vi "AutoBike FPGA.vi"() -> ()   [LabVIEW 2016]
doc: "The roboRIO FPGA Shipping Personality. This personality supports:\n- 8 Analog Input channels with 1 sample\n- 2 Analog Output channels with 1 sample\n- 30 Digital I/O channels with 1 sample\n- 1 RSL channel\n- 4 Relay channels\n- 1 Button\n- 3 LEDs\n- 1 Accelerometer\n- 13 PWM channels\n- 6 Encoder channels\n- 2 SPI channels\n- 2 I2C channels\n- 2 UART channels\n- 1 CAN channel\n- 2 Analog Input Interrupt\n- 5 Digital Input Interrupt\n- 1 Timer Interrupt"
uses:
  Sub VIs/Utilities/Start Boolean.ctl
  <vilib>/Platform/TimedLoop/XDataNode/timing_clust.ctl
  <vilib>/Platform/TimedLoop/XDataNode/nitl_modes.ctl
  <vilib>/Platform/TimedLoop/XDataNode/wakeup.ctl
  <vilib>/rvi/Emulation/niFpgaGetClockAttributes.vi
  <vilib>/rvi/Emulation/niFpgaSctlEmulationGetInTimedLoop.vi
  <vilib>/rvi/Emulation/niFpgaEmulationReportErrorSimple.vi
  <vilib>/rvi/eio/common/nirviEmuTemplateMethod_errors.vi
  <vilib>/rvi/Emulation/niFpgaCriticalErrorInLSC.vi
  <vilib>/rvi/Emulation/niFpgaProcessEmulError.vi
  <vilib>/rvi/Emulation/niFpgaEmulationIsFPGAContextNoSignature.vi
  <vilib>/rvi/errors/niFpgaSetErrorForExecOnDevCompSimple.vi
  <vilib>/rvi/eio/common/nirviEmuReportErrorAndStop.vi
  <vilib>/rvi/DataTransferAndStorage/Container/Common/niFpgaContainerGetUniqueNameForEmu.vi
  <vilib>/rvi/FIFO/Fifo_Resource/nirvififoEmulationSetSize.vi
  <vilib>/rvi/FIFO/Fifo_Resource/nirviFifoEmulationQueueMgr.vi
  <instcachedir>/0/nirviFifoEmulationQueueMgr_E5CAEC123FF24DC58D834DCA3CDAA9B5.lvgen/nirviFifoEmulationQueueMgr_E5CAEC123FF24DC58D834DCA3CDAA9B5_002.vi
  <vilib>/Utility/error.llb/Clear Errors.vi
  <vilib>/rvi/FIFO/Fifo_Resource/nirvififoEmulationCreateLock.vi
  <vilib>/rvi/FIFO/Fifo_Resource/nirvififoEmulationObtainLock.vi
  <vilib>/rvi/FIFO/Fifo_Resource/nirvififoEmulationReleaseLock.vi
  <vilib>/rvi/occurrence/nirviWaitOnOccurrenceBase.vi
  <vilib>/rvi/errors/nirviReportUnexpectedCaseInternalError.vi
  <vilib>/rvi/errors/nirviReportUnexpectedCaseInternalError (U32).vi
  <vilib>/rvi/FIFO/Fifo_Resource/nirvififoEmulationDetermineInputValidOut.vi
  <vilib>/rvi/DataTransferAndStorage/Container/Common/niFpgaContainerSetEmuInfo.vi
  <vilib>/eio/EIONode/EIONode.xnode
  <vilib>/rvi/DataTransferAndStorage/Container/XNode/niFpgaContainer.xnode
  <vilib>/rvi/FIFO/Fifo_Resource/nirvififoEmulationRead.vi
  <vilib>/rvi/FIFO/Fifo_Resource/nirvififoEmulationWrite.vi
  <vilib>/platform/TimedLoop/XDataNode/XDataNode.xnode
  <vilib>/rvi/LocalResourceManager/LocalResourceManager.xnode
  <vilib>/Platform/TimedLoop/XDataNode/XDNodeRunTimeDep.lvlib
panel:
  in  "Freq":u32 caption="Count(Ticks)"
  in  "Control Loop Duty Cycle":sgl
  in  "Control Loop Direction":bool
  in  "Front Panel Duty Cycle":sgl
  in  "Front Panel Direction":bool
  in  "Shut Down BW":bool
  out "Duty cycle (steering)":sgl
  out "Steering angle(deg)":sgl
  in  "Duty Cycle in":sgl
  in  "Count(uSec)":u32=1
  out "Current velocity":sgl
  out "Duty cycle (BW)":sgl
  in  "Reference velocity in km/h":sgl=15.0
  out "Filtered data":i32
  out "Value Channel 0":i32
  out "Channel 4 position":i32
  out "Channel 5 position":i32
  out "Channel 6 position":i32
  out "Channel 7 position":i32
  out "Position":i64
  in  "Stop encoder":bool
  in  "Reset counter":bool
  in  "Stop direction switch":bool
  in  "Switch direction":bool
  out "HallSensorValue":u8
  in  "Stop Hallsensor":bool
  out "dt":u32
  out "DIO.SPI_CS3:0.IN":u8 format="%08b"
  in  "DIO.SPI_CS3:0.DIR":u8 format="%08b"
  in  "DIO.SPI_CS3:0.OUT":u8 format="%08b"
  in  "IRQ.TIMER.SETTIME":T1
  in  "IRQ.TIMER.WRITE":u32
  out "IRQ.TIMER.READ":u32
  in  "IRQ.DI_BTN.NO":u8
  in  "IRQ.DI_BTN.CNT":u32
  in  "IRQ.DI_BTN.FALL":bool
  in  "IRQ.DI_BTN.RISE":bool
  in  "IRQ.DI_BTN.ENA":bool
  in  "IRQ.AI_B_0.HYSTERESIS":u16=17
  in  "IRQ.AI_B_1.HYSTERESIS":u16=17
  in  "IRQ.AI_B_1.NO":u8
  in  "IRQ.AI_B_0.NO":u8
  in  "IRQ.AI_B_1.THRESHOLD":u16
  in  "IRQ.AI_B_0.THRESHOLD":u16
  in  "IRQ.AI_B_3:0.CNFG":u8 format="%.0b"
  in  "IRQ.DIO_B_0.NO":u8
  in  "IRQ.DIO_B_1.NO":u8
  in  "IRQ.DIO_B_2.NO":u8
  in  "IRQ.DIO_B_3.NO":u8
  in  "IRQ.DIO_B_3.CNT":u32
  in  "IRQ.DIO_B_2.CNT":u32
  in  "IRQ.DIO_B_1.CNT":u32
  in  "IRQ.DIO_B_0.CNT":u32
  in  "IRQ.DIO_B_7:0.FALL":u8 format="%08b"
  in  "IRQ.DIO_B_7:0.RISE":u8 format="%08b"
  in  "IRQ.DIO_B_7:0.ENA":u8 format="%08b"
  in  "SPI.SPI.IRQ.NO":u8=15
  in  "SPI.B.IRQ.NO":u8=15
  out "DIO.DIO_9:8.IN":u8 format="%08b"
  in  "ENC.DIO_3.CNFG":u8 format="%08b"
  out "ENC.DIO_3.CNTR":u32
  out "ENC.DIO_3.STAT":u8 format="%08b"
  in  "ENC.DIO_4.CNFG":u8 format="%08b"
  out "ENC.DIO_4.CNTR":u32
  out "ENC.DIO_4.STAT":u8 format="%08b"
  in  "DIO.DIO_9:8.OUT":u8 format="%08b"
  in  "DIO.DIO_9:8.DIR":u8 format="%08b"
  in  "ENC.DIO_2.CNFG":u8 format="%08b"
  out "ENC.DIO_2.CNTR":u32
  out "ENC.DIO_2.STAT":u8 format="%08b"
  out "ENC.DIO_1.STAT":u8 format="%08b"
  out "ENC.DIO_1.CNTR":u32
  in  "ENC.DIO_1.CNFG":u8 format="%08b"
  out "DIO.DIO_7:0.IN":u8 format="%08b"
  in  "SYS.SELECTDIO":u8 format="%08b"
  in  "DIO.DIO_7:0.DIR":u8 format="%08b"
  in  "DIO.DIO_7:0.OUT":u8 format="%08b"
  out "ENC.DIO_0.STAT":u8 format="%08b"
  out "ENC.DIO_0.CNTR":u32
  in  "ENC.DIO_0.CNFG":u8 format="%08b"
  out "DI.BTN":u8 format="%08b"
  in  "DO.LED 5:0":u8 format="%06b"
  in  "DO.RSL.OUT":bool
  out "SPI.SPI.STAT":u8 format="%08b"
  in  "SPI.SPI.GO":T1
  in  "SPI.SPI.CNT":u16
  in  "SPI.SPI.CNFG":u16 format="%016b"
  out "SPI.SPI.DATI":u16
  in  "SPI.SPI.DATO":u16
  out "I2C.I2C.DATI":u8
  out "I2C.I2C.STAT":u8 format="%08b"
  in  "I2C.I2C.DATO":u8
  in  "I2C.I2CADDR":u8 format="%08b"
  in  "I2C.I2C.CNTR":u8
  in  "I2C.I2C.CNTL":u8 format="%08b"
  in  "I2C.I2C.CNFG":u8 format="%08b"
  in  "I2C.I2C.GO":T1
  out "ACC.Z.VAL":u16
  out "ACC.Y.VAL":u16
  out "ACC.X.VAL":u16
  in  "DO.RELAY.OUT":u8 format="%08b"
  out "SYS.ACC.RDY":bool
  out "SYS.RDY":bool
  in  "PWM.PWM_5.MAX":u16
  in  "PWM.PWM_5.CMP":u16
  in  "PWM.PWM_5.CNFG":u8 format="%08b"
  in  "PWM.PWM_5.CS":u8
  out "PWM.PWM_5.CNTR":u16
  in  "PWM.PWM_6.MAX":u16
  in  "PWM.PWM_6.CMP":u16
  in  "PWM.PWM_6.CNFG":u8 format="%08b"
  in  "PWM.PWM_6.CS":u8
  out "PWM.PWM_6.CNTR":u16
  in  "PWM.PWM_7.MAX":u16
  in  "PWM.PWM_7.CMP":u16
  in  "PWM.PWM_7.CNFG":u8 format="%08b"
  in  "PWM.PWM_7.CS":u8
  out "PWM.PWM_7.CNTR":u16
  in  "PWM.PWM_8.MAX":u16
  in  "PWM.PWM_8.CMP":u16
  in  "PWM.PWM_8.CNFG":u8 format="%08b"
  in  "PWM.PWM_8.CS":u8
  out "PWM.PWM_8.CNTR":u16
  in  "PWM.PWM_9.MAX":u16
  in  "PWM.PWM_9.CMP":u16
  in  "PWM.PWM_9.CNFG":u8 format="%08b"
  in  "PWM.PWM_9.CS":u8
  out "PWM.PWM_9.CNTR":u16
  in  "PWM.PWM_4.MAX":u16
  in  "PWM.PWM_4.CMP":u16
  in  "PWM.PWM_4.CNFG":u8 format="%08b"
  in  "PWM.PWM_4.CS":u8
  out "PWM.PWM_4.CNTR":u16
  in  "PWM.PWM_3.MAX":u16
  in  "PWM.PWM_3.CMP":u16
  in  "PWM.PWM_3.CNFG":u8 format="%08b"
  in  "PWM.PWM_3.CS":u8
  out "PWM.PWM_3.CNTR":u16
  in  "PWM.PWM_2.MAX":u16
  in  "PWM.PWM_2.CMP":u16
  in  "PWM.PWM_2.CNFG":u8 format="%08b"
  in  "PWM.PWM_2.CS":u8
  out "PWM.PWM_2.CNTR":u16
  in  "PWM.PWM_1.MAX":u16
  in  "PWM.PWM_1.CMP":u16
  in  "PWM.PWM_1.CNFG":u8 format="%08b"
  in  "PWM.PWM_1.CS":u8
  out "PWM.PWM_1.CNTR":u16
  out "PWM.PWM_0.CNTR":u16
  in  "PWM.PWM_0.CS":u8
  in  "PWM.PWM_0.CNFG":u8 format="%08b"
  in  "PWM.PWM_0.CMP":u16
  in  "PWM.PWM_0.MAX":u16
  in  "AO.B_0.VAL":u16
  in  "AO.B_1.VAL":u16
  in  "AO.SYS.GO":T1
  out "AO.SYS.STAT":bool
  out "AI.B_0.VAL":u16
  out "AI.B_1.VAL":u16
  out "AI.B_2.VAL":u16
  out "AI.B_3.VAL":u16
  out "AI.AI_0.VAL":u16
  out "AI.AI_1.VAL":u16
  out "AI.AI_2.VAL":u16
  out "AI.AI_3.VAL":u16
  out "SYS.AI.RDY":bool
  in  "SYS.SELECTB":u8 format="%08b"
  in  "DIO.B_7:0.OUT":u8 format="%08b"
  in  "DIO.B_7:0.DIR":u8 format="%08b"
  out "DIO.B_7:0.IN":u8 format="%08b"
  in  "DIO.B_15:8.OUT":u8 format="%08b"
  in  "DIO.B_15:8.DIR":u8 format="%08b"
  out "DIO.B_15:8.IN":u8 format="%08b"
  in  "SPI.B.DATO":u16
  out "SPI.B.DATI":u16
  in  "SPI.B.CNFG":u16 format="%016b"
  in  "SPI.B.CNT":u16
  in  "SPI.B.GO":T1
  out "SPI.B.STAT":u8 format="%08b"
  in  "PWM.B_0.MAX":u16
  in  "PWM.B_0.CMP":u16
  in  "PWM.B_0.CNFG":u8 format="%08b"
  in  "PWM.B_0.CS":u8
  out "PWM.B_0.CNTR":u16
  in  "PWM.B_1.CMP":u16
  in  "PWM.B_1.MAX":u16
  out "PWM.B_1.CNTR":u16
  in  "PWM.B_1.CNFG":u8 format="%08b"
  in  "PWM.B_1.CS":u8
  in  "PWM.B_2.CMP":u16
  in  "PWM.B_2.MAX":u16
  out "PWM.B_2.CNTR":u16
  in  "PWM.B_2.CNFG":u8 format="%08b"
  in  "PWM.B_2.CS":u8
  in  "I2C.B.DATO":u8
  out "I2C.B.DATI":u8
  in  "I2C.B.ADDR":u8 format="%08b"
  in  "I2C.B.CNTR":u8
  in  "I2C.B.CNTL":u8 format="%08b"
  out "I2C.B.STAT":u8 format="%08b"
  in  "I2C.B.CNFG":u8 format="%08b"
  in  "I2C.B.GO":T1
  in  "ENC.B.CNFG":u8 format="%08b"
  out "ENC.B.CNTR":u32
  out "ENC.B.STAT":u8 format="%08b"
  # "System"
  # "Onboard Devices"
  # "Connector B"
  # "DIO"
  # "SPI"
  # "PWM"
  # "I2C"
  # "AI"
  # "RELAY"
  # "RSL"
  # "Accelerometer"
  # "SPI Master"
  # "Analog Input"
  # "Analog Output"
  # "Digital I/O"
  # "Counters / PWM"
  # "Digital I/O"
  # "Encoders"
  # "IO Configuration"
  # "Buttons & LEDs"
  # "SPI CS DIO"
  # "Analog Interrupt"
  # "Digital Interrupt"
  # "Encoders"
  # "IO Configuration"
  # "Button Interrupt"
  # "I2C Master"
  # "FPGA Timer"
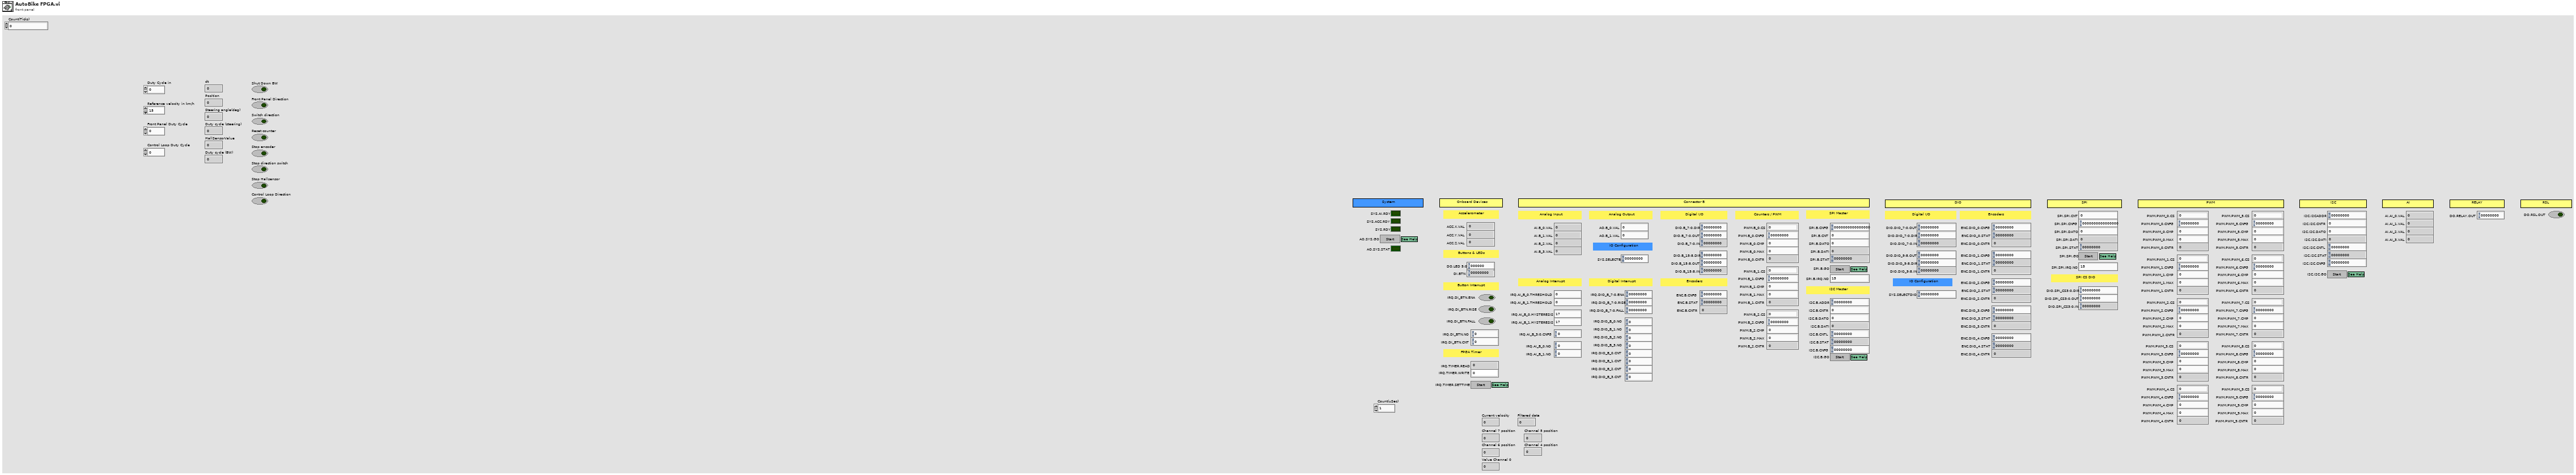
[diagram p1: front panel]
types:
  T1 = typedef "Start Boolean.ctl" = bool
  T2 = typedef "XDNodeRunTimeDep.lvlib/timing_clust.ctl" = cluster{"Expected End [f-1]":u64, "Actual End [f-1]":u64, "Finished Late? [f-1]":bool, "Expected End [i-1]":u64, "Actual End [i-1]":u64, "Finished Late? [i-1]":bool, "Expected Start [i]":u64, "Actual Start [i]":u64, "Expected Start [f]":u64, "Actual Start [f]":u64, "Source Name":string, "Structure Name":string, "Period":i64, "Deadline":i64, "Offset":i64, "Start":i64, "Priority":i32, "Timeout":i32, "Mode":T3, "Wakeup Reason":T4, "Error":errorcluster, "Source Type":string, "Secondary Source Type":string, "Global End Time":u64, "Global Start Time":u64, "Frame Duration":u64, "Iteration Duration":u64, "Assigned CPU":i32, "I/O Scan Engine Mode":u32}
  T3 = typedef "XDNodeRunTimeDep.lvlib/nitl_modes.ctl" = enum32{"No Change", "Process missed periods, maintain original phase", "Discard missed periods, maintain original phase", "Process missed periods, ignore original phase", "Discard missed periods, ignore original phase"}
  T4 = typedef "XDNodeRunTimeDep.lvlib/wakeup.ctl" = enum32{"Normal", "Aborted", "Asynchronous wakeup", "Timing source error", "Timed loop error", "Timeout"}
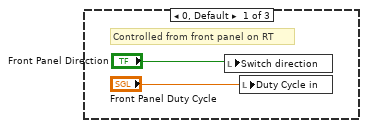
[diagram p2: hidden frame]
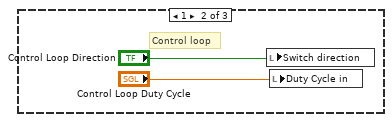
[diagram p3: hidden frame]
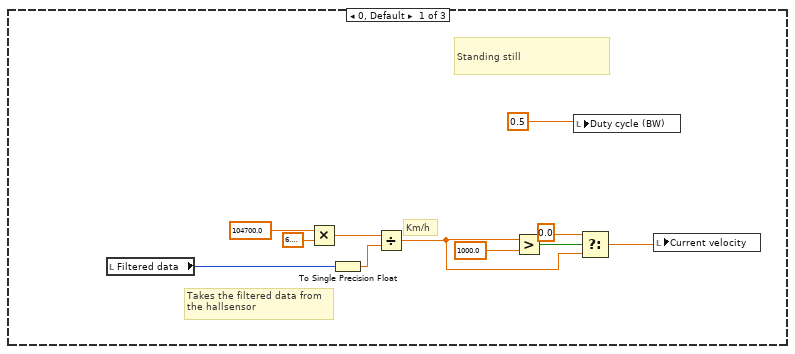
[diagram p4: hidden frame]
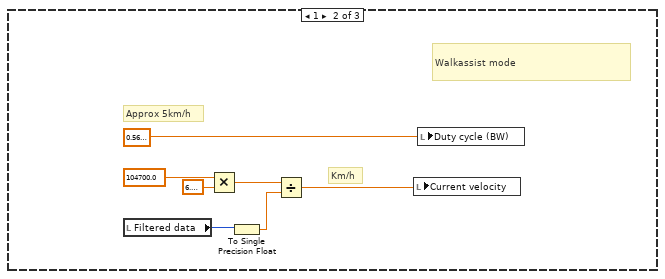
[diagram p5: hidden frame]
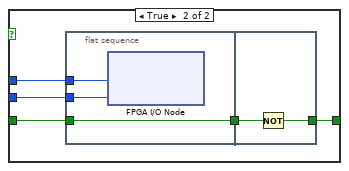
[diagram p12: hidden frame]
diagram:
  # "DONT USE PWN 1, IT IS CONNECTED ON THREE OUTS"
  # "The accelerometer nodes take some time before the FPGA can first read the values. This is because it takes time to read from the accelerometer. An iteration of the While Loop will not complete until the accelerometer values have been read.\n\nAfter the completion of the first iteration of the While Loop, all indicators have valid values."
  # "The analog output nodes take some time before the FPGA write the values to the pins. The GO and STAT registers are used to handshake between the FPGA and host. When the host wants the values to be written, the host sets the GO register to TRUE. If the host reads the STAT register before setting the value of the GO register, it can wait for the value of the STAT register to invert. The value inversion tells the host that the output values have been written."
  # "The FPGA timer fires the interrupt request (IRQ) when TIMER.Read counts down to zero. If TIMER.Read is not zero, it counts down to one per microsecond."
  # "The analog input nodes take some time before the FPGA can first read the values. This is because it takes time to set up the Analog-to-Digital converter (ADC) and convert the first reading. An iteration of the While Loop will not complete until all the analog input channels have been sampled.\n\nAfter the completion of the first iteration of the While Loop, all indicators have valid values."
  # "Note: On some hardware a \"ghosting effect\" may occur on any unconnected AI channels. For example, if channel AI0 is connected and channels AI1~AI7 are not connected the the value read at AI0 may be seen on indicators AI1~AI7. This is common for hardware that use a multiplexed (MUXed) Analog-to-Digital converter (ADC), because the input analog signal is used to charge a capacitor which does not discharge before the unconnected channel is read.\n\nYou can hide the \"ghosting effect\" by using an mask register. This register is used to decide when the indicator should be updated."
  # "The only interface that sends interrupts to the RT side. Timer interrupts, analog input interrupts, digital input interrupts, and SPI interrupt share this interface.\n\nAll interrupts work in sequence. One interrupt waits until the previous interrupt request (IRQ) gets acknowledged on the RT side."
  # "NOTE: The SYS.RDY boolean MUST exist and must become TRUE at some point otherwise the myRIO API will not function correctly."
  # "There is some delay between when the FPGA code starts and the analog inputs, accelerometer, and scaling values outputs are valid. If the host wants to ensure that there are valid values in theses registers it should wait for each subsystem to finish its initialization process. \n\nWhen all subsystems have finished initializinig, the SYS.RDY indicator will be true, which can be polled by the host to determine the status of the FPGA. Alternatively, the host can poll the individual SYS.xx.RDY indicators to determine the status of the individual subsystems.\n\nThis loop continues indefinitely, essentially making SYS.RDY a read-only register."
  n1 = flat-sequence {
    tunnel: [i64 0] -> w2
    tunnel: [TRUE ("DIO/DIO3")] -> w1
    tunnel: w2 -> [w29]
    tunnel: w1 -> [w28]
    frame #0 {
      # "Initialise"
    }
    frame #1 {
      n2 = while {
        shift-right: [w49] -> _
        shift-left: w28 -> [w51]
        stop <- "Stop Hallsensor" stop-if-true
        n3 = flat-sequence {
          tunnel: w51 -> [w54]
          tunnel: [w54] -> w48
          tunnel: [u8 0] -> w47
          tunnel: [w52] -> w46
          tunnel: w48 -> [w59]
          tunnel: w47 -> [w57]
          tunnel: w46 -> [w56]
          tunnel: [w58] -> w45
          tunnel: [w55] -> w44
          tunnel: [w81] -> w49
          tunnel: w45 -> [w81]
          tunnel: [w80] -> w43
          tunnel: w44 -> [w78]
          frame #0 {
            n4 = call "Tick Count4"() -> ("Tick Count(uSec)"=w52:u32)
          }
          frame #1 {
            n5 = node-c288() -> (w61:T2)  [unwired: 1 in]
            n6 = timed-loop {
              shift-right: [w65] -> _
              shift-left: w57 -> [w62]
              shift-right: [w70] -> w58
              shift-left: w59 -> [w73]
              timing: w61 -> [_]
              timing-out: [_] -> w60
              tunnel: w56 -> [w72]
              tunnel: [w72] -> w55
              stop <- w64 stop-if-true
              # "Calculates the time it takes to collect 2 rises, i.e one magnet"
              # "Reads the output from the hallsensor and outputs the number of change in rises"
              # "Hallsensor counter"
              n7 = xnode "FPGA I/O Node"() -> ("DIO/DIO8"=w70:bool)  [unwired: 1 in, 1 out]
              n8 = Exclusive Or(1:w73, 2:w70) -> (0:w68:bool)
              n9 = Not And(1:TRUE ("y"), 2:w70) -> (0:w69:bool)
              n10 = And(x=w69, y=w68) -> (x .and. y?=w67:bool)
              n11 = Increment(x=w62) -> (x+1=w66:u8)
              n12 = Select(t=w66, s=w67, f=w62) -> (s? t:f=w65:u8)
              "HallSensorValue" <- w65
              n13 = Equal?(x=u8 2, y=w65) -> (x = y?=w64:bool)
            }
            n14 = node-c288(w60) -> ()
          }
          frame #2 {
            n15 = call "Tick Count"() -> ("Tick Count(uSec)"=w79:u32)
            n16 = Subtract(x=w79, y=w78) -> (x-y=w80:u32)
          }
        }
        n17 = To Long Integer(number=w43) -> (32bit integer=w42:i32)
        n18 = call "Median filter.vi"("Rawdata"=w42) -> ("Filtered element"=w39:i32)  [unwired: 10 in]
        n19 = Equal To 0?(x=w39) -> (x = 0?=w41:bool)
        n20 = Select(t=1, s=w41, f=w39) -> (s? t:f=→"Filtered data":i32)
      }
      n21 = node-c288() -> (w31:T2)  [unwired: 1 in]
      n22 = node-c288() -> (w27:T2)  [unwired: 1 in]
      n23 = timed-loop {
        shift-right: [w92] -> _
        shift-left: w29 -> [w83]
        shift-right: [w89] -> _
        shift-left: _ -> [w87]
        shift-right: [w88] -> _
        shift-left: _ -> [w86]
        timing: w31 -> [_]
        timing-out: [_] -> w30
        stop <- "Stop encoder" stop-if-true
        # "Decoder, reads both signals and check if there is any change to any of the channels, if there is a change current A channel\nis compared to previous B channel to determine which direction the motor is going and updates the position counter\naccordingly. The counter is resetted each time the Main VI is deployed."
        # "Motor Decoder"
        n24 = xnode "FPGA I/O Node"() -> ("DIO/DIO0"=w89:bool, "DIO/DIO1"=w88:bool)  [unwired: 2 in, 2 out]
        n25 = Exclusive Or(1:w86, 2:w89) -> (0:w85:bool)
        n26 = Select(t=i64 0, s="Reset counter", f=w83) -> (s? t:f=w91:i64)
        n27 = Exclusive Or(1:w87, 2:w89) -> (0:w99:bool)
        n28 = Exclusive Or(1:w86, 2:w88) -> (0:w98:bool)
        n29 = Or(x=w99, y=w98) -> (x .or. y?=w84:bool)
        n30 = Select(t=i64 1, s=w85, f=i64 -1) -> (s? t:f=w94:i64)
        n31 = Add(x=w94, y=w91) -> (x+y=w93:i64)
        n32 = Select(t=w93, s=w84, f=w91) -> (s? t:f=w92:i64)
        "Position" <- w92
      }
      n33 = timed-loop {
        timing: w27 -> [_]
        timing-out: [_] -> w26
        stop <- "Stop direction switch" stop-if-true
        # "Switch the direction of the steering\nmotor."
        # "Switch direction"
        n34 = xnode "FPGA I/O Node"("DIO/DIO2"="Switch direction") -> ()  [unwired: 1 in, 1 out]
      }
      n35 = node-c288(w26) -> ()
      n36 = node-c288(w30) -> ()
    }
  }
  n37 = while {
    stop <- FALSE stop-if-true
    # "PWM signal to steering motor"
    n38 = flat-sequence {
      tunnel: ["Freq"] -> w104
      tunnel: [w112] -> w106
      tunnel: w104 -> [w109]
      tunnel: w106 -> [w114]
      frame #0 {
        # "2000 ticks=20 000Hz"
        n39 = call "Loop Timer3"("Count(Ticks)"="Freq") -> ()  [unwired: 1 out]
      }
      frame #1 {
        n40 = local read "Duty cycle (steering)"() -> (w110:sgl)
        n41 = To Single Precision Float(number=w109) -> (single precision float=w108:sgl)
        n42 = Not Equal To 0?(x=w110) -> (x != 0?=w111:bool)
        n43 = Multiply(x=w110, y=w108) -> (x*y=w113:sgl)
        n44 = xnode "FPGA I/O Node"("PWM/PWM0"=w111) -> ()  [unwired: 1 in, 1 out]
        n45 = To Unsigned Long Integer(number=w113) -> (unsigned 32bit integer=w112:u32)
      }
      frame #2 {
        n46 = call "Wait3"("Count(Ticks)"=w114) -> ()  [unwired: 1 out]
      }
      frame #3 {
        n47 = xnode "FPGA I/O Node"("PWM/PWM0"=FALSE ("PWM/PWM8")) -> ()  [unwired: 1 in, 1 out]
      }
    }
  }
  n48 = while {
    stop <- FALSE stop-if-true
    # "Backwheel motor control"
    n49 = local read "Channel 5 position"() -> (w116:i32)
    n50 = case shown="2" w116 {
      frame 0, Default {
        # "Takes the filtered data from\nthe hallsensor"
        # "Km/h"
        # "Standing still"
        n51 = local read "Filtered data"() -> (w119:i32)
        n52 = Multiply(x=sgl 104700.0, y=sgl 6.2831855) -> (x*y=w125:sgl)
        n53 = To Single Precision Float(number=w119) -> (single precision float=w120:sgl)
        n54 = Divide(x=w125, y=w120) -> (x/y=w121:sgl)
        n55 = Greater?(x=w121, y=sgl 1000.0) -> (0:w123:bool)
        n56 = local write "Duty cycle (BW)"(sgl 0.5 ("Duty cycle out 2")) -> ()
        n57 = Select(t=sgl 0.0, s=w123, f=w121) -> (s? t:f=w118:sgl)
        n58 = local write "Current velocity"(w118) -> ()
      }
      frame 1 {
        # "Walkassist mode"
        # "Approx 5km/h"
        # "Km/h"
        n59 = local read "Filtered data"() -> (w132:i32)
        n60 = Multiply(x=sgl 104700.0, y=sgl 6.2831855) -> (x*y=w133:sgl)
        n61 = To Single Precision Float(number=w132) -> (single precision float=w131:sgl)
        n62 = Divide(x=w133, y=w131) -> (x/y=w130:sgl)
        n63 = local write "Current velocity"(w130) -> ()
        n64 = local write "Duty cycle (BW)"(sgl 0.56 ("Duty cycle out")) -> ()
      }
      frame 2 {
        n65 = while {
          shift-right: [w141] -> _
          shift-left: sgl 0.56 -> [w144]
          stop <- w138 stop-if-true
          # "This is in case we are starting from\nstanding still and we try to divide with 0, \nwhich will give us an inf value."
          # "Cruise control"
          # "Takes the filtered data from\nthe hallsensor"
          # "Wheel radius=0.349m\nnumber of magnets=12\nFormulas:\ndt/1 000 000 * number of magnets = time between magnets\nDivide wheel circumfence with time between two magnets multiplied\n by number of magnets, multiplied by 3.6 to get it in km/h.\n\n(2pi(0.349*1 000 000*3.6/12)) / dt = km/h"
          # "Km/h"
          n66 = local read "Filtered data"() -> (w150:i32)
          n67 = Multiply(x=sgl 104700.0, y=sgl 6.2831855) -> (x*y=w156:sgl)
          n68 = To Single Precision Float(number=w150) -> (single precision float=w151:sgl)
          n69 = Divide(x=w156, y=w151) -> (x/y=w152:sgl)
          n70 = Greater?(x=w152, y=sgl 1000.0) -> (0:w154:bool)
          n71 = Select(t=sgl 0.0, s=w154, f=w152) -> (s? t:f=w137:sgl)
          "Current velocity" <- w137
          n72 = Less Or Equal?(x=w137, y="Reference velocity in km/h") -> (x <= y?=w142:bool)
          n73 = Add(x=sgl 1e-06 ("y"), y=w144) -> (x+y=w145:sgl)
          n74 = Subtract(x=w144, y=sgl 1e-06) -> (x-y=w146:sgl)
          n75 = local read "Channel 5 position"() -> (w140:i32)
          n76 = Select(t=w145, s=w142, f=w146) -> (s? t:f=w141:sgl)
          "Duty cycle (BW)" <- w141
          n77 = call "Wait"("Count(uSec)"="Count(uSec)") -> ()  [unwired: 1 out]
          n78 = Not Equal?(x=w140, y=2) -> (x != y?=w138:bool)
        }
      }
    }
  }
  n79 = while {
    stop <- FALSE stop-if-true
    # "PWM signal to backwheel motor"
    n80 = flat-sequence {
      tunnel: [w164] -> w160
      tunnel: w160 -> [w167]
      frame #0 {
        # "80 000ticks=500Hz"
        n81 = call "Loop Timer2"("Count(Ticks)"=u32 80000) -> ()  [unwired: 1 out]
      }
      frame #1 {
        n82 = local read "Duty cycle (BW)"() -> (w162:sgl)
        n83 = xnode "FPGA I/O Node"("PWM/PWM8"=TRUE) -> ()  [unwired: 1 in, 1 out]
        n84 = Multiply(x=w162, y=sgl 80000.0) -> (x*y=w165:sgl)
        n85 = To Unsigned Long Integer(number=w165) -> (unsigned 32bit integer=w164:u32)
      }
      frame #2 {
        n86 = call "Wait2"("Count(Ticks)"=w167) -> ()  [unwired: 1 out]
      }
      frame #3 {
        n87 = xnode "FPGA I/O Node"("PWM/PWM8"=FALSE) -> ()  [unwired: 1 in, 1 out]
      }
    }
  }
  n88 = while {
    stop <- FALSE stop-if-true
    # "Host Synchronization"
    n89 = local read "SYS.ACC.RDY"() -> (w170:bool)
    n90 = local read "SYS.AI.RDY"() -> (w172:bool)
    n91 = Compound Arithmetic op=AND(w172, w170) -> (→"SYS.RDY":bool)
  }
  n92 = while {
    stop <- FALSE stop-if-true
    # "Interrupt to RT"
    n93 = xnode ("FIFO Method Node")("Timeout"=-1) -> ("Element"=w175:u8)  [unwired: 1 in, 2 out]
    n94 = call <vilib>:"niFPGA Interrupt.vi"("Wait Until Cleared (F)"=TRUE, "IRQ Number (0)"=w175) -> ()  [unwired: 1 in]
  }
  n95 = while {
    stop <- FALSE stop-if-true
    # "Steering motor"
    n96 = local read "Switch direction"() -> (w182:bool)
    n97 = local read "Position"() -> (w179:i64)
    n98 = call "Steering motor.vi"("Steering position (in pulses)"=w179, "Duty Cycle in"="Duty Cycle in", "Switch direction"=w182) -> ("Duty Cycle out"=→"Duty cycle (steering)":sgl, "Steering angle(deg)"=→"Steering angle(deg)":sgl)  [unwired: 7 in]
  }
  n99 = while {
    stop <- FALSE stop-if-true
    # "Receiver"
    n100 = call "Receiver.vi"() -> ("Channel 7 position"=→"Channel 7 position":i32, "Channel 6 position"=→"Channel 6 position":i32, "Channel 5 position"=w186:i32, "Channel 4 position"=→"Channel 4 position":i32, "Value Channel 0"=→"Value Channel 0":i32)  [unwired: 7 in]
    n101 = Select(t=0, s="Shut Down BW", f=w186) -> (s? t:f=→"Channel 5 position":i32)
  }
  n102 = while {
    stop <- FALSE stop-if-true
    # "RC steering motor switch"
    n103 = local read "Channel 6 position"() -> (w193:i32)
    n104 = case shown="2" w193 {
      frame 0, Default {
        # "Controlled from front panel on RT"
        n105 = local write "Switch direction"("Front Panel Direction") -> ()
        n106 = local write "Duty Cycle in"("Front Panel Duty Cycle") -> ()
      }
      frame 1 {
        # "Control loop"
        n107 = local write "Switch direction"("Control Loop Direction") -> ()
        n108 = local write "Duty Cycle in"("Control Loop Duty Cycle") -> ()
      }
      frame 2 {
        n109 = local read "Value Channel 0"() -> (w200:i32)
        n110 = call "RC steering motor interpolation.vi"("Value Channel 0"=w200) -> ("Numeric"=w199:sgl, "Boolean"=w198:bool)  [unwired: 9 in]
        n111 = local write "Duty Cycle in"(w199) -> ()
        n112 = local write "Switch direction"(w198) -> ()
      }
    }
  }
  n113 = while {
    stop <- FALSE stop-if-true
    # "Timer"
    n114 = local read "IRQ.TIMER.READ"() -> (w204:u32)
    n115 = Select(t="IRQ.TIMER.WRITE", s="IRQ.TIMER.SETTIME", f=w204) -> (s? t:f=w202:u32)
    n116 = case shown="Default" w202 {
      selector: w202 -> [w208 w211]
      tunnel: [w208 w209] -> w201
      frame 0 {
      }
      frame Default {
        n117 = Decrement(x=w211) -> (x-1=w210:u32)
        n118 = case shown="0" w210 {
          selector: w210 -> [w212 w215]
          tunnel: [w212 w215] -> w209
          frame Default {
          }
          frame 0 {
            w214 = u8 0  # Reserved for Timer IRQ
            n119 = xnode ("FIFO Method Node")("Element"=w214, "Timeout"=-1) -> ()  [unwired: 1 in, 2 out]
          }
        }
      }
    }
    "IRQ.TIMER.READ" <- w201
    n120 = call "Loop Timer"("Count(uSec)"=u8 1 ("Count(mSec)")) -> ()  [unwired: 1 out]
  }
  n121 = xnode "VI-Defined FIFO Configuration"() -> ("FIFO Out"=w4:refnum<k21>)
  n122 = while {
    tunnel: w4 -> [w224]
    i -> [w238]
    stop <- FALSE stop-if-true
    # "Analog Input"
    n123 = Greater Than 0?(x=w238) -> (x > 0?=→"SYS.AI.RDY":bool)
    n124 = xnode "FPGA I/O Node"() -> ("MXP/AI0"=w217:u16, "MXP/AI1"=w216:u16, "MXP/AI2"=→"AI.B_2.VAL":u16, "MXP/AI3"=→"AI.B_3.VAL":u16, "AnalogIn0"=→"AI.AI_0.VAL":u16, "AnalogIn1"=→"AI.AI_1.VAL":u16, "AnalogIn2"=→"AI.AI_2.VAL":u16, "AnalogIn3"=→"AI.AI_3.VAL":u16)  [unwired: 8 in, 8 out]
    "AI.B_0.VAL" <- w217
    "AI.B_1.VAL" <- w216
    n125 = Number To Boolean Array(number="IRQ.AI_B_3:0.CNFG") -> (Boolean array=w225:bool[])
    n126 = Index Array(array=w225) -> (element #1=w227:bool, element #2=w228:bool, element #3=w230:bool, element #4=w231:bool)  [unwired: 4 in]
    n127 = call "Check AI IRQ.vi"("Hysteresis"="IRQ.AI_B_1.HYSTERESIS", "FIFO In"=w224, "IRQ Number"="IRQ.AI_B_1.NO", "Threshold"="IRQ.AI_B_1.THRESHOLD", "Analog Value"=w216, "Rising Edge?"=w231, "Enable Interrupt?"=w230) -> ()  [unwired: 5 in]
    n128 = call "Check AI IRQ.vi"("Hysteresis"="IRQ.AI_B_0.HYSTERESIS", "FIFO In"=w224, "IRQ Number"="IRQ.AI_B_0.NO", "Threshold"="IRQ.AI_B_0.THRESHOLD", "Analog Value"=w217, "Rising Edge?"=w228, "Enable Interrupt?"=w227) -> ()  [unwired: 5 in]
  }
  n129 = while {
    stop <- FALSE stop-if-true
    # "Analog Output"
    n130 = feedback #1(FALSE) -> (w242:bool)
    n131 = case shown="False" "AO.SYS.GO" {
      tunnel: "AO.B_0.VAL" -> [_ w252]
      tunnel: "AO.B_1.VAL" -> [_ w251]
      tunnel: w242 -> [w247 w250]
      tunnel: [w247 w248] -> w240
      frame False {
      }
      frame True {
        n132 = flat-sequence {
          tunnel: w252 -> [w255]
          tunnel: w251 -> [w254]
          tunnel: w250 -> [w253]
          tunnel: [w253] -> w249
          tunnel: w249 -> [w257]
          tunnel: [w256] -> w248
          frame #0 {
            n133 = xnode "FPGA I/O Node"("MXP/AO0"=w255, "MXP/AO1"=w254) -> ()  [unwired: 2 in, 2 out]
          }
          frame #1 {
            n134 = Not(x=w257) -> (.not. x?=w256:bool)
          }
        }
      }
    }
    "AO.SYS.STAT" <- w240
    n135 = feedback-in #1(w240) -> ()
  }
  n136 = while {
    i -> [w265]
    stop <- FALSE stop-if-true
    # "Onboard Accelerometer"
    n137 = xnode "FPGA I/O Node"() -> ("AccelerationX"=w263:i16, "AccelerationY"=w262:i16, "AccelerationZ"=w261:i16)  [unwired: 3 in, 3 out]
    n138 = Greater Than 0?(x=w265) -> (x > 0?=→"SYS.ACC.RDY":bool)
    n139 = To Unsigned Word Integer(number=w263) -> (unsigned 16bit integer=→"ACC.X.VAL":u16)
    n140 = To Unsigned Word Integer(number=w262) -> (unsigned 16bit integer=→"ACC.Y.VAL":u16)
    n141 = To Unsigned Word Integer(number=w261) -> (unsigned 16bit integer=→"ACC.Z.VAL":u16)
  }
  n142 = xnode "VI-Defined FIFO Configuration"() -> ("FIFO Out"=w3:refnum<k21>)
  n143 = node-c288() -> (w9:T2)  [unwired: 1 in]
  n144 = timed-loop {
    timing: w9 -> [_]
    timing-out: [_] -> w8
    tunnel: w3 -> [w272]
    stop <- FALSE stop-if-true
    # "Button IRQ"
    # "Onboard DIO"
    n145 = xnode "FPGA I/O Node"() -> ("User Button"=w273:bool)  [unwired: 1 in, 1 out]
    n146 = Number To Boolean Array(number="DO.LED 5:0") -> (Boolean array=w283:bool[])
    n147 = Index Array(array=w283) -> (element #1=w281:bool, element #2=w280:bool, element #3=w279:bool, element #4=w278:bool, element #5=w277:bool, element #6=w276:bool)  [unwired: 6 in]
    n148 = Build Array(w273) -> (w275:bool[])
    n149 = call "DIO IRQ 1-bit.vi"("IRQ.NO"="IRQ.DI_BTN.NO", "IRQ.CNT"="IRQ.DI_BTN.CNT", "FIFO in"=w272, "IRQ.FALL"="IRQ.DI_BTN.FALL", "IRQ.RISE"="IRQ.DI_BTN.RISE", "IRQ.ENA"="IRQ.DI_BTN.ENA", "DIO"=w273) -> ()  [unwired: 5 in]
    n150 = Boolean Array To Number(Boolean array=w275) -> (number=→"DI.BTN":u8)
    n151 = xnode "FPGA I/O Node"("Radio LED Green"=w281, "Radio LED Red"=w280, "Comm LED Green"=w279, "Comm LED Red"=w278, "Mode LED Green"=w277, "Mode LED Red"=w276) -> ()  [unwired: 6 in, 6 out]
  }
  n152 = while {
    stop <- FALSE stop-if-true
    # "Button SCTL Interrupt Buffer"
    n153 = feedback #2(u8 0 ("Element")) -> (w289:u8)
    n154 = feedback #3(FALSE ("Timed Out?")) -> (w293:bool)
    n155 = case shown="False" w293 {
      tunnel: [w295 w297] -> w290
      tunnel: w289 -> [_ w297]
      frame False {
        n156 = xnode ("FIFO Read")("Timeout"=-1) -> ("Element"=w295:u8)  [unwired: 1 in, 2 out]
      }
      frame True {
      }
    }
    n157 = feedback-in #2(w290) -> ()
    n158 = xnode ("FIFO Method Node")("Element"=w290, "Timeout"=0) -> ("Timed Out?"=w291:bool)  [unwired: 1 in, 1 out]
    n159 = feedback-in #3(w291) -> ()
  }
  n160 = node-c288(w8) -> ()
  n161 = xnode "VI-Defined FIFO Configuration"() -> ("FIFO Out"=w7:refnum<k21>)
  n162 = xnode "VI-Defined FIFO Configuration"() -> ("FIFO Out"=w5:refnum<k21>)
  n163 = node-c288() -> (w23:T2)  [unwired: 1 in]
  n164 = timed-loop {
    timing: w23 -> [_]
    timing-out: [_] -> w22
    tunnel: w7 -> [w334]
    tunnel: w5 -> [w322]
    stop <- _ stop-if-true
    # "DIO/ IRQ"
    # "DIO / Encoder"
    # "DIO / I2C Master"
    # "DIO / PWM"
    # "DIO"
    # "DIO"
    # "DIO/ SPI Master"
    # "Connector MXP DIO"
    n165 = call "Split HDC Bank1 DIO.vi"("IN 7:0"="DIO.B_7:0.OUT") -> ("OUT 3:0"=w422:fxp<+,4,4>, "OUT 4"=w337:bool, "OUT 7:5"=w419:fxp<+,3,3>)
    n166 = call "Split HDC Bank1 DIO.vi"("IN 7:0"="DIO.B_7:0.DIR") -> ("OUT 3:0"=w421:fxp<+,4,4>, "OUT 4"=w420:bool, "OUT 7:5"=w418:fxp<+,3,3>)
    n167 = call "Split HDC Function Select.vi"("IN 7:0"="SYS.SELECTB") -> ("OUT 1:0"=w358:fxp<+,2,2>, "OUT 7"=w353:bool, "OUT 2"=w357:bool, "OUT 3"=w356:bool, "OUT 4"=w355:bool, "OUT 5"=w354:bool)
    n168 = call "DIO 4-bit.vi"("DIO0 Refnum"=refnum<k21> "MXP/DIO0", "DIO1 Refnum"=refnum<k21> "MXP/DIO1", "DIO2 Refnum"=refnum<k21> "MXP/DIO2", "DIR 3:0"=w421, "OUT 3:0"=w422, "DIO3 Refnum"=refnum<k21> "MXP/DIO3") -> ("IN 3:0"=w333:fxp<+,4,4>)  [unwired: 5 in]
    n169 = call "DIO 1-bit.vi"("DIR"=w420, "OUT"=w337, "DIO Refnum"=refnum<k21> "MXP/DIO4") -> ("IN"=w394:bool)  [unwired: 8 in]
    n170 = call "DIO_SPI.vi"("DIO.2:0.OUT"=w419, "DIO.2:0.DIR"=w418, "SPI.CNT"="SPI.B.CNT", "SPI.CNFG"="SPI.B.CNFG", "SPI.DATO"="SPI.B.DATO", "SPI.GO"="SPI.B.GO", "DIO.2/SPI.MOSI Refnum"=refnum<k21> "MXP/DIO7" ("DIO.2/SPI.SCLK"), "SELECT.1:0"=w358, "DIO.1/SPI.MISO Refnum"=refnum<k21> "MXP/DIO6" ("DIO.1/SPI.MOSI"), "DIO.0/SPI.SCLK Refnum"=refnum<k21> "MXP/DIO5" ("DIO.0/SPI.MISO")) -> ("DIO.2:0.IN"=w393:fxp<+,3,3>, "SPI.DATI"=→"SPI.B.DATI":u16, "SPI.STAT"=w336:u8)  [unwired: 7 in]
    "SPI.B.STAT" <- w336
    n171 = call "SPI IRQ.vi"("SPI.A.IRQ.NO"="SPI.B.IRQ.NO", "SPI.STAT"=w336, "FIFO In"=w334) -> ()  [unwired: 9 in]
    n172 = call "Join HDC Bank1 DIO.vi"("IN 7:5"=w393, "IN 4"=w394, "IN 3:0"=w333) -> ("OUT 7:0"=→"DIO.B_7:0.IN":u8)
    n173 = Number To Boolean Array(number="IRQ.DIO_B_7:0.ENA") -> (Boolean array=w319:bool[])
    n174 = Number To Boolean Array(number="IRQ.DIO_B_7:0.RISE") -> (Boolean array=w310:bool[])
    n175 = Number To Boolean Array(number="IRQ.DIO_B_7:0.FALL") -> (Boolean array=w305:bool[])
    n176 = Index Array(array=w319) -> (element #1=w320:bool, element #2=w318:bool, element #3=w317:bool, element #4=w316:bool)  [unwired: 4 in]
    n177 = Index Array(array=w310) -> (element #1=w309:bool, element #2=w311:bool, element #3=w312:bool, element #4=w313:bool)  [unwired: 4 in]
    n178 = Index Array(array=w305) -> (element #1=w306:bool, element #2=w304:bool, element #3=w303:bool, element #4=w302:bool)  [unwired: 4 in]
    n179 = Build Array(w320, w318, w317, w316) -> (w321:bool[])
    n180 = Build Array(w309, w311, w312, w313) -> (w308:bool[])
    n181 = Build Array(w306, w304, w303, w302) -> (w307:bool[])
    n182 = Build Array("IRQ.DIO_B_0.CNT", "IRQ.DIO_B_1.CNT", "IRQ.DIO_B_2.CNT", "IRQ.DIO_B_3.CNT") -> (w328:u32[])
    n183 = Build Array("IRQ.DIO_B_0.NO", "IRQ.DIO_B_1.NO", "IRQ.DIO_B_2.NO", "IRQ.DIO_B_3.NO") -> (w323:u8[])
    n184 = Boolean Array To Number(Boolean array=w321) -> (number=w314:fxp<+,4,4>)
    n185 = Boolean Array To Number(Boolean array=w308) -> (number=w299:fxp<+,4,4>)
    n186 = Boolean Array To Number(Boolean array=w307) -> (number=w298:fxp<+,4,4>)
    n187 = call "DIO IRQ 4-bit.vi"("IRQ NO"=w323, "IRQ CNT"=w328, "FIFO In"=w322, "IRQ.FALL"=w298, "IRQ.RISE"=w299, "IRQ.ENA"=w314, "IN 3:0"=w333) -> ()  [unwired: 5 in]
    n188 = call "Split HDC Bank2 DIO.vi"("IN 7:0"="DIO.B_15:8.OUT") -> ("OUT 5"=w339:bool, "OUT 7:6"=w363:fxp<+,2,2>, "OUT 4:3"=w341:fxp<+,2,2>, "OUT 2"=w343:bool, "OUT 0"=w347:bool, "OUT 1"=w346:bool)  [unwired: 2 in]
    n189 = call "Split HDC Bank2 DIO.vi"("IN 7:0"="DIO.B_15:8.DIR") -> ("OUT 5"=w338:bool, "OUT 7:6"=w362:fxp<+,2,2>, "OUT 4:3"=w340:fxp<+,2,2>, "OUT 2"=w342:bool, "OUT 0"=w345:bool, "OUT 1"=w344:bool)  [unwired: 2 in]
    n190 = call "DIO_PWM.vi"("DIO.OUT"=w347, "DIO.DIR"=w345, "PWM.CS"="PWM.B_0.CS", "PWM.CNFG"="PWM.B_0.CNFG", "PWM.CMP"="PWM.B_0.CMP", "PWM.MAX"="PWM.B_0.MAX", "DIO/PWM"=refnum<k21> "MXP/DIO8", "SELECT"=w357) -> ("DIO.IN"=w352:bool, "PWM.CNTR"=→"PWM.B_0.CNTR":u16)  [unwired: 10 in]
    n191 = call "DIO_PWM.vi"("DIO.OUT"=w346, "DIO.DIR"=w344, "PWM.CS"="PWM.B_1.CS", "PWM.CNFG"="PWM.B_1.CNFG", "PWM.CMP"="PWM.B_1.CMP", "PWM.MAX"="PWM.B_1.MAX", "DIO/PWM"=refnum<k21> "MXP/DIO9", "SELECT"=w356) -> ("DIO.IN"=w351:bool, "PWM.CNTR"=→"PWM.B_1.CNTR":u16)  [unwired: 10 in]
    n192 = call "DIO_PWM.vi"("DIO.OUT"=w343, "DIO.DIR"=w342, "PWM.CS"="PWM.B_2.CS", "PWM.CNFG"="PWM.B_2.CNFG", "PWM.CMP"="PWM.B_2.CMP", "PWM.MAX"="PWM.B_2.MAX", "DIO/PWM"=refnum<k21> "MXP/DIO10", "SELECT"=w355) -> ("DIO.IN"=w350:bool, "PWM.CNTR"=→"PWM.B_2.CNTR":u16)  [unwired: 10 in]
    n193 = call "DIO_Encoder.vi"("DIO.1:0.OUT"=w341, "DIO.1:0.DIR"=w340, "QE.CNFG"="ENC.B.CNFG", "DIO.1/QE.B"=refnum<k21> "MXP/DIO12", "SELECT"=w354, "DIO.0/QE.A"=refnum<k21> "MXP/DIO11") -> ("DIO.1:0.IN"=w349:fxp<+,2,2>, "QE.CNTR"=→"ENC.B.CNTR":u32, "QE.STAT"=→"ENC.B.STAT":u8)  [unwired: 11 in]
    n194 = call "DIO 1-bit.vi"("DIR"=w338, "OUT"=w339, "DIO Refnum"=refnum<k21> "MXP/DIO13") -> ("IN"=w348:bool)  [unwired: 8 in]
    n195 = call "DIO_I2C.vi"("DIO.1:0.OUT"=w363, "DIO.1:0.DIR"=w362, "I2C.CNFG"="I2C.B.CNFG", "I2C.CNTL"="I2C.B.CNTL", "I2C.ADDR"="I2C.B.ADDR", "I2C.DATO"="I2C.B.DATO", "DIO.1/I2C.SDA"=refnum<k21> "MXP/DIO15" ("DIO.1/I2C.SCL"), "I2C.CNTR"="I2C.B.CNTR", "DIO.0/I2C.SCL"=refnum<k21> "MXP/DIO14" ("DIO.0/I2C.SDA"), "Execute?"="I2C.B.GO", "SELECT"=w353) -> ("DIO.1:0.IN"=w360:fxp<+,2,2>, "I2C.DATI"=→"I2C.B.DATI":u8, "I2C.STAT"=→"I2C.B.STAT":u8)  [unwired: 6 in]
    n196 = call "Join HDC Bank2 DIO.vi"("IN 7:6"=w360, "IN 5"=w348, "IN 4:3"=w349, "IN 0"=w352, "IN 2"=w350, "IN 1"=w351) -> ("OUT 7:0"=→"DIO.B_15:8.IN":u8)  [unwired: 4 in]
  }
  n197 = while {
    stop <- FALSE stop-if-true
    # "Connector A SPI SCTL Interrupt Buffer"
    n198 = feedback #4(u8 0 ("Element")) -> (w427:u8)
    n199 = feedback #5(FALSE ("Timed Out?")) -> (w431:bool)
    n200 = case shown="False" w431 {
      tunnel: [w433 w435] -> w428
      tunnel: w427 -> [_ w435]
      frame False {
        n201 = xnode ("FIFO Method Node")("Timeout"=-1) -> ("Element"=w433:u8)  [unwired: 1 in, 2 out]
      }
      frame True {
      }
    }
    n202 = feedback-in #4(w428) -> ()
    n203 = xnode ("FIFO Method Node")("Element"=w428, "Timeout"=0) -> ("Timed Out?"=w429:bool)  [unwired: 1 in, 1 out]
    n204 = feedback-in #5(w429) -> ()
  }
  n205 = while {
    stop <- FALSE stop-if-true
    # "Connector A DIO SCTL Interrupt Buffer"
    n206 = feedback #6(u8 0 ("Element")) -> (w438:u8)
    n207 = feedback #7(FALSE ("Timed Out?")) -> (w442:bool)
    n208 = case shown="False" w442 {
      tunnel: [w444 w446] -> w439
      tunnel: w438 -> [_ w446]
      frame False {
        n209 = xnode ("FIFO Method Node")("Timeout"=-1) -> ("Element"=w444:u8)  [unwired: 1 in, 2 out]
      }
      frame True {
      }
    }
    n210 = feedback-in #6(w439) -> ()
    n211 = xnode ("FIFO Method Node")("Element"=w439, "Timeout"=0) -> ("Timed Out?"=w440:bool)  [unwired: 1 in, 1 out]
    n212 = feedback-in #7(w440) -> ()
  }
  n213 = node-c288(w22) -> ()
  n214 = node-c288() -> (w17:T2)  [unwired: 1 in]
  n215 = timed-loop {
    timing: w17 -> [_]
    timing-out: [_] -> w16
    stop <- FALSE stop-if-true
    # "Detta ska vara dio4"
    # "DIO"
    n216 = call "Split HDC Bank3 DIO.vi"("IN 7:0"="DIO.DIO_7:0.OUT") -> ("OUT 1:0"=w462:fxp<+,2,2>, "OUT 3:2"=w461:fxp<+,2,2>, "OUT 5:4"=w460:fxp<+,2,2>, "OUT 7:6"=w452:fxp<+,2,2>)
    n217 = call "Split HDC Bank3 DIO.vi"("IN 7:0"="DIO.DIO_7:0.DIR") -> ("OUT 1:0"=w458:fxp<+,2,2>, "OUT 3:2"=w457:fxp<+,2,2>, "OUT 5:4"=w456:fxp<+,2,2>, "OUT 7:6"=w451:fxp<+,2,2>)
    n218 = Number To Boolean Array(number="SYS.SELECTDIO") -> (Boolean array=w493:bool[])
    n219 = Index Array(array=w493) -> (element #1=w492:bool, element #2=w489:bool, element #3=w480:bool, element #4=w469:bool, element #5=w468:bool)  [unwired: 5 in]
    n220 = call "DIO_Encoder.vi"("DIO.1:0.OUT"=w452, "DIO.1:0.DIR"=w451, "QE.CNFG"="ENC.DIO_3.CNFG", "DIO.1/QE.B"=refnum<k21> "DIO/DIO7" ("DIO Refnum"), "SELECT"=w469, "DIO.0/QE.A"=refnum<k21> "DIO/DIO6" ("DIO Refnum")) -> ("DIO.1:0.IN"=w450:fxp<+,2,2>, "QE.CNTR"=→"ENC.DIO_3.CNTR":u32, "QE.STAT"=→"ENC.DIO_3.STAT":u8)  [unwired: 11 in]
    n221 = call "DIO_Encoder.vi"("DIO.1:0.OUT"=w462, "DIO.1:0.DIR"=w458, "QE.CNFG"="ENC.DIO_0.CNFG", "DIO.1/QE.B"=refnum<k21> "DIO/DIO1" ("DIO Refnum"), "SELECT"=w492, "DIO.0/QE.A"=refnum<k21> "DIO/DIO0" ("DIO Refnum")) -> ("DIO.1:0.IN"=w467:fxp<+,2,2>, "QE.CNTR"=→"ENC.DIO_0.CNTR":u32, "QE.STAT"=→"ENC.DIO_0.STAT":u8)  [unwired: 11 in]
    n222 = call "DIO_Encoder.vi"("DIO.1:0.OUT"=w461, "DIO.1:0.DIR"=w457, "QE.CNFG"="ENC.DIO_1.CNFG", "DIO.1/QE.B"=refnum<k21> "DIO/DIO3" ("DIO Refnum"), "SELECT"=w489, "DIO.0/QE.A"=refnum<k21> "DIO/DIO2" ("DIO Refnum")) -> ("DIO.1:0.IN"=w466:fxp<+,2,2>, "QE.CNTR"=→"ENC.DIO_1.CNTR":u32, "QE.STAT"=→"ENC.DIO_1.STAT":u8)  [unwired: 11 in]
    n223 = call "DIO_Encoder.vi"("DIO.1:0.OUT"=w460, "DIO.1:0.DIR"=w456, "QE.CNFG"="ENC.DIO_2.CNFG", "DIO.1/QE.B"=refnum<k21> "DIO/DIO5" ("DIO Refnum"), "SELECT"=w480, "DIO.0/QE.A"=refnum<k21> "DIO/DIO2" ("DIO Refnum")) -> ("DIO.1:0.IN"=w465:fxp<+,2,2>, "QE.CNTR"=→"ENC.DIO_2.CNTR":u32, "QE.STAT"=→"ENC.DIO_2.STAT":u8)  [unwired: 11 in]
    n224 = call "Join HDC Bank3 DIO.vi"("IN 7:6"=w450, "IN 5:4"=w465, "IN 3:2"=w466, "IN 1:0"=w467) -> ("OUT 7:0"=→"DIO.DIO_7:0.IN":u8)
    n225 = call "Split HDC Bank3 DIO.vi"("IN 7:0"="DIO.DIO_9:8.OUT") -> ("OUT 1:0"=w449:fxp<+,2,2>)  [unwired: 3 out]
    n226 = call "Split HDC Bank3 DIO.vi"("IN 7:0"="DIO.DIO_9:8.DIR") -> ("OUT 1:0"=w448:fxp<+,2,2>)  [unwired: 3 out]
    n227 = call "DIO_Encoder.vi"("DIO.1:0.OUT"=w449, "DIO.1:0.DIR"=w448, "QE.CNFG"="ENC.DIO_4.CNFG", "DIO.1/QE.B"=refnum<k21> "DIO/DIO9" ("DIO Refnum"), "SELECT"=w468, "DIO.0/QE.A"=refnum<k21> "DIO/DIO8" ("DIO Refnum")) -> ("DIO.1:0.IN"=w447:fxp<+,2,2>, "QE.CNTR"=→"ENC.DIO_4.CNTR":u32, "QE.STAT"=→"ENC.DIO_4.STAT":u8)  [unwired: 11 in]
    n228 = call "Join HDC Bank3 DIO.vi"("IN 1:0"=w447) -> ("OUT 7:0"=→"DIO.DIO_9:8.IN":u8)  [unwired: 3 in]
  }
  n229 = node-c288(w16) -> ()
  n230 = node-c288() -> (w21:T2)  [unwired: 1 in]
  n231 = timed-loop {
    timing: w21 -> [_]
    timing-out: [_] -> w20
    stop <- FALSE stop-if-true
    # "PWM1 were PWM8"
    # "First PWM1 were PWM0"
    # "PWM"
    n232 = call "PWM (Single Output).vi"("Clock Select"="PWM.PWM_0.CS", "Counter Control"="PWM.PWM_0.CNFG", "Output Compare Value"="PWM.PWM_0.CMP", "Max Counter Value"="PWM.PWM_0.MAX") -> ("Output"=w558:bool, "Counter Value"=→"PWM.PWM_0.CNTR":u16)  [unwired: 6 in]
    n233 = call "PWM (Single Output).vi"("Clock Select"="PWM.PWM_1.CS", "Counter Control"="PWM.PWM_1.CNFG", "Output Compare Value"="PWM.PWM_1.CMP", "Max Counter Value"="PWM.PWM_1.MAX") -> ("Output"=w552:bool, "Counter Value"=→"PWM.PWM_1.CNTR":u16)  [unwired: 6 in]
    n234 = call "PWM (Single Output).vi"("Clock Select"="PWM.PWM_2.CS", "Counter Control"="PWM.PWM_2.CNFG", "Output Compare Value"="PWM.PWM_2.CMP", "Max Counter Value"="PWM.PWM_2.MAX") -> ("Output"=w536:bool, "Counter Value"=→"PWM.PWM_2.CNTR":u16)  [unwired: 6 in]
    n235 = call "PWM (Single Output).vi"("Clock Select"="PWM.PWM_3.CS", "Counter Control"="PWM.PWM_3.CNFG", "Output Compare Value"="PWM.PWM_3.CMP", "Max Counter Value"="PWM.PWM_3.MAX") -> ("Output"=w535:bool, "Counter Value"=→"PWM.PWM_3.CNTR":u16)  [unwired: 6 in]
    n236 = call "PWM (Single Output).vi"("Clock Select"="PWM.PWM_4.CS", "Counter Control"="PWM.PWM_4.CNFG", "Output Compare Value"="PWM.PWM_4.CMP", "Max Counter Value"="PWM.PWM_4.MAX") -> ("Output"=w534:bool, "Counter Value"=→"PWM.PWM_4.CNTR":u16)  [unwired: 6 in]
    n237 = xnode "FPGA I/O Node"("PWM/PWM1"=w558, "PWM/PWM1"=w552, "PWM/PWM2"=w536, "PWM/PWM3"=w535, "PWM/PWM4"=w534) -> ()  [unwired: 5 in, 5 out]
    n238 = call "PWM (Single Output).vi"("Clock Select"="PWM.PWM_5.CS", "Counter Control"="PWM.PWM_5.CNFG", "Output Compare Value"="PWM.PWM_5.CMP", "Max Counter Value"="PWM.PWM_5.MAX") -> ("Output"=w509:bool, "Counter Value"=→"PWM.PWM_5.CNTR":u16)  [unwired: 6 in]
    n239 = call "PWM (Single Output).vi"("Clock Select"="PWM.PWM_6.CS", "Counter Control"="PWM.PWM_6.CNFG", "Output Compare Value"="PWM.PWM_6.CMP", "Max Counter Value"="PWM.PWM_6.MAX") -> ("Output"=w515:bool, "Counter Value"=→"PWM.PWM_6.CNTR":u16)  [unwired: 6 in]
    n240 = call "PWM (Single Output).vi"("Clock Select"="PWM.PWM_7.CS", "Counter Control"="PWM.PWM_7.CNFG", "Output Compare Value"="PWM.PWM_7.CMP", "Max Counter Value"="PWM.PWM_7.MAX") -> ("Output"=w531:bool, "Counter Value"=→"PWM.PWM_7.CNTR":u16)  [unwired: 6 in]
    n241 = call "PWM (Single Output).vi"("Clock Select"="PWM.PWM_8.CS", "Counter Control"="PWM.PWM_8.CNFG", "Output Compare Value"="PWM.PWM_8.CMP", "Max Counter Value"="PWM.PWM_8.MAX") -> ("Output"=w532:bool, "Counter Value"=→"PWM.PWM_8.CNTR":u16)  [unwired: 6 in]
    n242 = call "PWM (Single Output).vi"("Clock Select"="PWM.PWM_9.CS", "Counter Control"="PWM.PWM_9.CNFG", "Output Compare Value"="PWM.PWM_9.CMP", "Max Counter Value"="PWM.PWM_9.MAX") -> ("Output"=w533:bool, "Counter Value"=→"PWM.PWM_9.CNTR":u16)  [unwired: 6 in]
    n243 = xnode "FPGA I/O Node"("PWM/PWM5"=w509, "PWM/PWM6"=w515, "PWM/PWM7"=w531, "PWM/PWM1"=w532, "PWM/PWM9"=w533) -> ()  [unwired: 5 in, 5 out]
  }
  n244 = node-c288(w20) -> ()
  n245 = xnode "VI-Defined FIFO Configuration"() -> ("FIFO Out"=w6:refnum<k21>)
  n246 = node-c288() -> (w13:T2)  [unwired: 1 in]
  n247 = timed-loop {
    timing: w13 -> [_]
    timing-out: [_] -> w12
    tunnel: w6 -> [w568]
    stop <- FALSE stop-if-true
    # "SPI / CS DIO"
    # "SPI / SPI"
    # "SPI"
    n248 = xnode "FPGA I/O Node"() -> ("SPI MISO"=w585:bool)  [unwired: 1 in, 1 out]
    n249 = call "SPI Master.vi"("Count"="SPI.SPI.CNT", "Configuration"="SPI.SPI.CNFG", "Start?"="SPI.SPI.GO", "MISO"=w585, "Data Out"="SPI.SPI.DATO") -> ("Status"=w566:u8, "SCLK"=w579:bool, "MOSI"=w580:bool, "Data In"=→"SPI.SPI.DATI":u16)  [unwired: 3 in]
    "SPI.SPI.STAT" <- w566
    n250 = xnode "FPGA I/O Node"("SPI MOSI"=w580, "SPI CLK"=w579) -> ()  [unwired: 2 in, 2 out]
    n251 = call "SPI IRQ.vi"("SPI.A.IRQ.NO"="SPI.SPI.IRQ.NO", "SPI.STAT"=w566, "FIFO In"=w568) -> ()  [unwired: 9 in]
    n252 = call "Split HDC Bank1 DIO.vi"("IN 7:0"="DIO.SPI_CS3:0.OUT") -> ("OUT 3:0"=w575:fxp<+,4,4>)  [unwired: 2 out]
    n253 = call "Split HDC Bank1 DIO.vi"("IN 7:0"="DIO.SPI_CS3:0.DIR") -> ("OUT 3:0"=w574:fxp<+,4,4>)  [unwired: 2 out]
    n254 = call "DIO 4-bit.vi"("DIO0 Refnum"=refnum<k21> "SPI CS0", "DIO1 Refnum"=refnum<k21> "SPI CS1" ("DIO0 Refnum"), "DIO2 Refnum"=refnum<k21> "SPI CS2" ("DIO0 Refnum"), "DIR 3:0"=w574, "OUT 3:0"=w575, "DIO3 Refnum"=refnum<k21> "SPI CS3" ("DIO0 Refnum")) -> ("IN 3:0"=w573:fxp<+,4,4>)  [unwired: 5 in]
    n255 = call "Join HDC Bank1 DIO.vi"("IN 3:0"=w573) -> ("OUT 7:0"=→"DIO.SPI_CS3:0.IN":u8)  [unwired: 2 in]
  }
  n256 = while {
    stop <- FALSE stop-if-true
    # "Connector SPI SPI SCTL Interrupt Buffer"
    n257 = feedback #8(u8 0 ("Element")) -> (w592:u8)
    n258 = feedback #9(FALSE ("Timed Out?")) -> (w596:bool)
    n259 = case shown="False" w596 {
      tunnel: [w598 w600] -> w593
      tunnel: w592 -> [_ w600]
      frame False {
        n260 = xnode ("FIFO Method Node")("Timeout"=-1) -> ("Element"=w598:u8)  [unwired: 1 in, 2 out]
      }
      frame True {
      }
    }
    n261 = feedback-in #8(w593) -> ()
    n262 = xnode ("FIFO Method Node")("Element"=w593, "Timeout"=0) -> ("Timed Out?"=w594:bool)  [unwired: 1 in, 1 out]
    n263 = feedback-in #9(w594) -> ()
  }
  n264 = node-c288(w12) -> ()
  n265 = node-c288() -> (w15:T2)  [unwired: 1 in]
  n266 = timed-loop {
    timing: w15 -> [_]
    timing-out: [_] -> w14
    stop <- FALSE stop-if-true
    # "I2C"
    n267 = call "DIO_I2C.vi"("I2C.CNFG"="I2C.I2C.CNFG", "I2C.CNTL"="I2C.I2C.CNTL", "I2C.ADDR"="I2C.I2CADDR", "I2C.DATO"="I2C.I2C.DATO", "DIO.1/I2C.SDA"=refnum<k21> "I2C SDA" ("FPGA I/O In"), "I2C.CNTR"="I2C.I2C.CNTR", "DIO.0/I2C.SCL"=refnum<k21> "I2C SCL" ("FPGA I/O In"), "Execute?"="I2C.I2C.GO", "SELECT"=TRUE) -> ("I2C.DATI"=→"I2C.I2C.DATI":u8, "I2C.STAT"=→"I2C.I2C.STAT":u8)  [unwired: 8 in, 1 out]
  }
  n268 = node-c288(w14) -> ()
  n269 = node-c288() -> (w19:T2)  [unwired: 1 in]
  n270 = timed-loop {
    timing: w19 -> [_]
    timing-out: [_] -> w18
    stop <- FALSE stop-if-true
    # "Relay"
    n271 = Number To Boolean Array(number="DO.RELAY.OUT") -> (Boolean array=w623:bool[])
    n272 = Index Array(array=w623) -> (element #1=w622:bool, element #2=w621:bool, element #3=w620:bool, element #4=w619:bool, element #5=w618:bool, element #6=w617:bool, element #7=w616:bool, element #8=w615:bool)  [unwired: 8 in]
    n273 = xnode "FPGA I/O Node"("RelayFwd0"=w622, "RelayRev0"=w621, "RelayFwd1"=w620, "RelayRev1"=w619, "RelayFwd2"=w618, "RelayRev2"=w617, "RelayFwd3"=w616, "RelayRev3"=w615) -> ()  [unwired: 8 in, 8 out]
  }
  n274 = node-c288(w18) -> ()
  n275 = node-c288() -> (w11:T2)  [unwired: 1 in]
  n276 = timed-loop {
    timing: w11 -> [_]
    timing-out: [_] -> w10
    stop <- FALSE stop-if-true
    # "RSL"
    n277 = xnode "FPGA I/O Node"("RSL"="DO.RSL.OUT") -> ()  [unwired: 1 in, 1 out]
  }
  n278 = node-c288(w10) -> ()
